vi "DurationToMB.vi"(1 "Experiment Duration (hr)":dbl=20.0, 2 "fs (hz)":u16) -> (0 "FileSize(MB)":i16)   [LabVIEW 2020]
doc: "computes file size (MB) to allocate for SD card based on sampling rate, test duration.\nImportant: Update BYTES_PER_DATA_FRAME accordingly. As of June 19 2019, there are 286 bytes in each data frame (each scan)"
panel:
  in  "BYTES_PER_DATA_FRAME":dbl=286.0 format="%#_13g"
  # "FOR 128CH SYSTEM JUNE 19 2019"
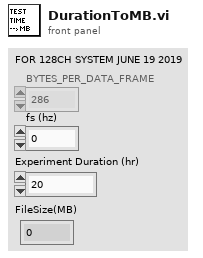
[diagram p1: front panel]
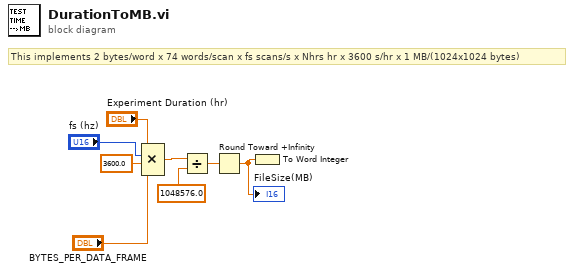
[diagram p0: block diagram]
diagram:
  # "This implements 2 bytes/word x 74 words/scan x fs scans/s x Nhrs hr x 3600 s/hr x 1 MB/(1024x1024 bytes)"
  n1 = Compound Arithmetic op=MULTIPLY("Experiment Duration (hr)", "fs (hz)", 3600.0 ("value"), "BYTES_PER_DATA_FRAME") -> (w5:dbl)
  n2 = Divide(x=w5, y=1048576.0) -> (x/y=w3:dbl)
  n3 = Round Toward +Infinity(x=w3) -> (ceil(x): smallest int >= x=w2:dbl)
  "FileSize(MB)" <- w2
  n4 = To Word Integer(number=w2) -> ()  [unwired: 1 out]
